vi "Set Options.vi"(8 "error in (no error)":errorcluster, 10 "Initial Options (Empty)":string[](array[string]), 11 "AutoComplete in":refnum<class "AutoComplete.lvclass">) -> (0 "error out":errorcluster, 3 "AutoComplete out":refnum<class "AutoComplete.lvclass">)   [LabVIEW 2020, in "AutoComplete.lvlib" / "AutoComplete.lvclass"]
doc: "Specifies a new list of options that should be available in the autocomplete. This can be useful for filtering out already selected items (See the Selected List Demo example) or updating the list when application state changes."
uses:
  AutoComplete.lvclass
  AutoComplete.lvclass/AutoComplete.ctl
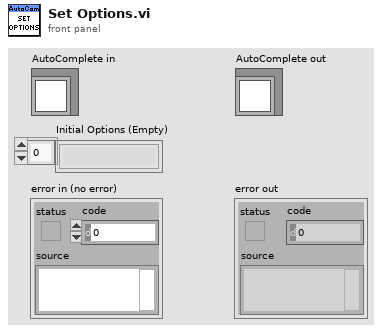
[diagram p1: front panel]
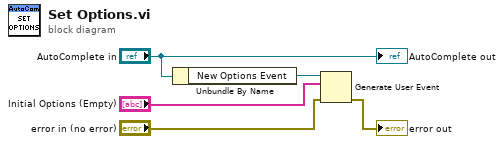
[diagram p0: block diagram]
diagram:
  n1 = Unbundle By Name("AutoComplete in") -> ("New Options Event"=w4:refnum<user-event>)
  n2 = Generate User Event(user event=w4, event data cluster="Initial Options (Empty)", error in="error in (no error)") -> (error out=→"error out":errorcluster)  [unwired: 1 in, 1 out]
  "AutoComplete out" <- "AutoComplete in"
